vi "Configure Session.vi"(8 "error in":errorcluster, 11 "Plugin in":refnum<class "StreamReader.lvclass">) -> (0 "error out":errorcluster, 3 "Plugin out":refnum<class "StreamReader.lvclass">)   [LabVIEW 2024, in "StreamReader.lvlib" / "StreamReader.lvclass"]
uses:
  StreamReader.lvclass
  C:/Program Files/National Instruments/LabVIEW 2024/vi.lib/FlexLogger/SDK/PluginSDK.lvlibp/PEFClasses/SDK/Plugin/Plugin.lvclass
  StreamReader.lvclass/StreamReader.ctl
  StreamReader Strings.vi
  <vilib>/FlexLogger/SDK/PluginSDK.lvlibp/PEFClasses/SDK/Plugin/ParameterAccess/Read String.vi
  <vilib>/FlexLogger/SDK/PluginSDK.lvlibp/PEFClasses/SDK/Plugin/ParameterAccess/Read I32.vi
  <vilib>/FlexLogger/SDK/PluginSDK.lvlibp/PEFClasses/SDK/Plugin/Plugin.lvclass
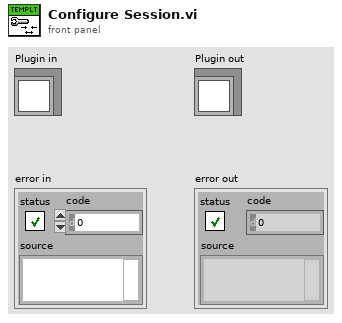
[diagram p1: front panel]
types:
  T1 = typedef "StreamReader.lvlib/StreamReader.lvclass/StreamReader Parameters.ctl" = cluster{"Reader URL":string, "Writer URL":string, "Timeout":i32, "Buffer Size":i32, "Reader endpoint":refnum<k21>, "Channel Names":string[]}
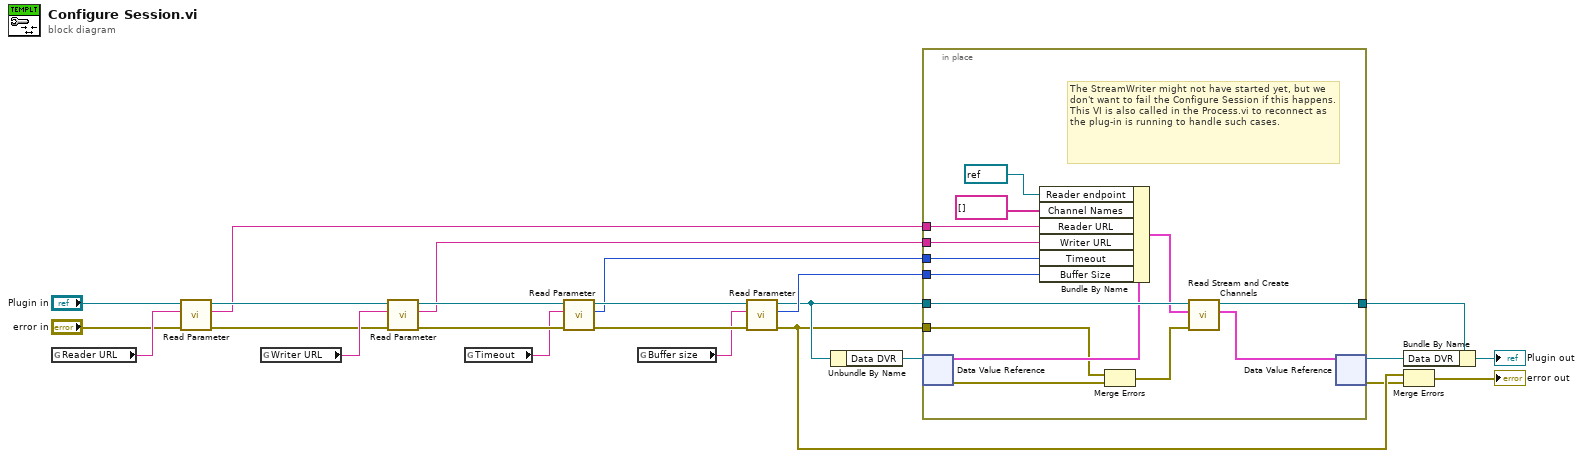
[diagram p0: block diagram]
diagram:
  n1 = global read "StreamReader Strings.vi" "Reader URL"() -> (w12:string)
  n2 = call-poly <vilib>:"Read Parameter.vi"("error in (no error)"="error in", "Name"=w12, "Plugin in"="Plugin in") -> ("error out"=w8:errorcluster, "Value"=w7:string, "Plugin out"=w10:refnum<class "StreamReader.lvclass">)  [unwired: 5 in, 1 out]
  n3 = global read "StreamReader Strings.vi" "Writer URL"() -> (w20:string)
  n4 = call-poly <vilib>:"Read Parameter.vi"("error in (no error)"=w8, "Name"=w20, "Plugin in"=w10) -> ("error out"=w22:errorcluster, "Value"=w15:string, "Plugin out"=w24:refnum<class "StreamReader.lvclass">)  [unwired: 5 in, 1 out]
  n5 = global read "StreamReader Strings.vi" "Timeout"() -> (w19:string)
  n6 = call-poly <vilib>:"Read Parameter.vi"("error in (no error)"=w22, "Name"=w19, "Plugin in"=w24) -> ("error out"=w21:errorcluster, "Value"=w14:i32, "Plugin out"=w23:refnum<class "StreamReader.lvclass">)  [unwired: 5 in, 1 out]
  n7 = global read "StreamReader Strings.vi" "Buffer size"() -> (w18:string)
  n8 = call-poly <vilib>:"Read Parameter.vi"("error in (no error)"=w21, "Name"=w18, "Plugin in"=w23) -> ("error out"=w3:errorcluster, "Value"=w16:i32, "Plugin out"=w6:refnum<class "StreamReader.lvclass">)  [unwired: 5 in, 1 out]
  n9 = Unbundle By Name(w6) -> ("Data DVR"=w5:refnum<data-value>)
  n10 = in-place {
    in-place-border: w16 -> [w38]
    in-place-border: w15 -> [w37]
    in-place-border: w14 -> [w36]
    in-place-border: w6 -> [w35]
    in-place-border: [w33] -> w13
    in-place-border: w3 -> [w28]
    in-place-border: w7 -> [w32]
    # "The StreamWriter might not have started yet, but we don't want to fail the Configure Session if this happens.\nThis VI is also called in the Process.vi to reconnect as the plug-in is running to handle such cases."
    n11 = in-place-dvr #1(w5) -> (w31:T1, w29:errorcluster)
    n12 = Bundle By Name(cluster=w31, "Reader endpoint"=refnum<k21> refnum, "Channel Names"=string[] [], "Reader URL"=w32, "Writer URL"=w37, "Timeout"=w36, "Buffer Size"=w38) -> (w34:T1)
    n13 = Merge Errors(w28, w29) -> (w27:errorcluster)
    n14 = call-dynamic "Read Stream and Create Channels.vi"("error in (no error)"=w27, "StreamReader Parameters in"=w34, "Plugin in"=w35) -> ("StreamReader Parameters out"=w30:T1, "Plugin out"=w33:refnum<class "StreamReader.lvclass">)  [unwired: 5 in, 2 out]
    n15 = in-place-dvr #1(w30) -> (w4:refnum<data-value>, w2:errorcluster)
  }
  n16 = Bundle By Name(cluster=w13, "Data DVR"=w4) -> (→"Plugin out":refnum<class "StreamReader.lvclass">)
  n17 = Merge Errors(w3, w2) -> (→"error out":errorcluster)
